vi "Teardown.vi"(8 "error in (no error)":errorcluster, 11 "LUnit Test Runner Test In":refnum<class "Test Runner Test.lvclass">) -> (0 "error out":errorcluster, 3 "LUnit Test Runner Test Out":refnum<class "Test Runner Test.lvclass">)   [LabVIEW 2020, in "Test Runner Test.lvclass"]
uses:
  Test Runner Test.lvclass
  Test Runner Test.lvclass/Test Runner Test.ctl
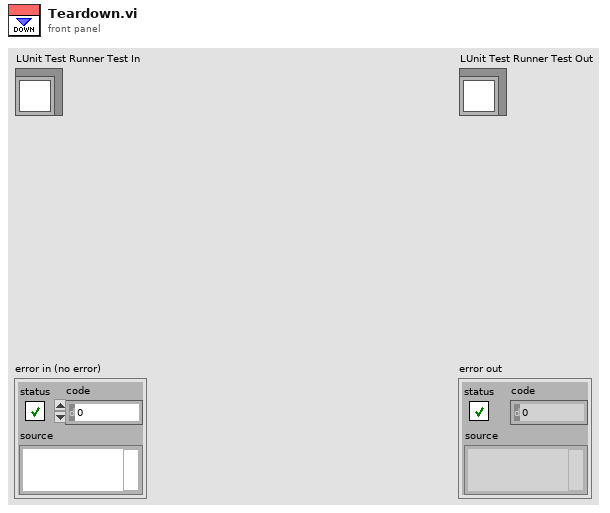
[diagram p1: front panel]
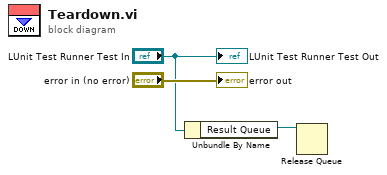
[diagram p0: block diagram]
diagram:
  n1 = Unbundle By Name("LUnit Test Runner Test In") -> ("Result Queue"=w1:refnum<queue>)
  n2 = Release Queue(queue=w1) -> ()  [unwired: 2 in, 3 out]
  "error out" <- "error in (no error)"
  "LUnit Test Runner Test Out" <- "LUnit Test Runner Test In"
